vi "Html Title Exchange.vi"(8 "font":T3={"font name"="", "font size"=0.0, "bold"=0, "italic"=0, "underline"=0, "strike through"=0, "font color"=16777216} {"font size" format="%0.2f"; "strike through" items=["Strk Unchanged", "Strk Yes", "Strk No"]; "underline" items=["Und Unchanged", "Und Yes", "Und No"]; "italic" items=["Ital Unchanged", "Ital Yes", "Ital No"]; "bold" items=["Bold Unchanged", "Bold Yes", "Bold No"]}) -> (0 "text color (unchanged)":u32(colorbox)=16777216, 2 "font settings":T2={"Charset (-1)"=-1, "Weight (-1)"=-1, "Name"="", "Size"=" "}, 3 "text options":T1)   [LabVIEW 2014]
uses:
  <vilib>/addons/_office/_wordsub.llb/font.ctl
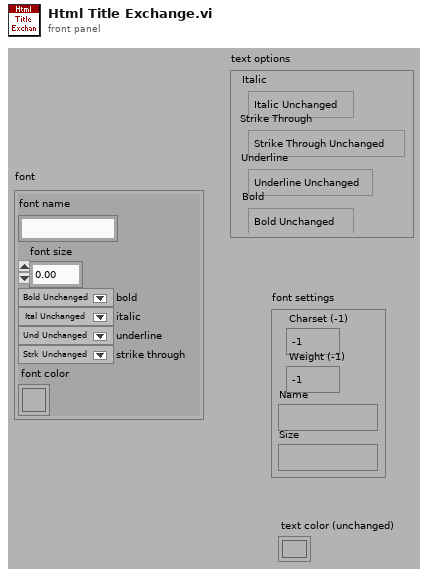
[diagram p1: front panel]
types:
  T1 = cluster{"Italic":enum16{"Italic Unchanged", "Italic On", "Italic Off"}, "Strike Through":enum16{"Strike Through Unchanged", "Strike Through On", "Strike Through Off"}, "Underline":enum16{"Underline Unchanged", "Underline On", "Underline Off"}, "Bold":enum16{"Bold Unchanged", "Bold On", "Bold Off"}}
  T2 = cluster{"Charset (-1)":i16, "Weight (-1)":i16, "Name":string, "Size":string}
  T3 = typedef "font.ctl" = cluster{"font name":string, "font size":dbl, "bold":u16, "italic":u16, "underline":u16, "strike through":u16, "font color":u32}
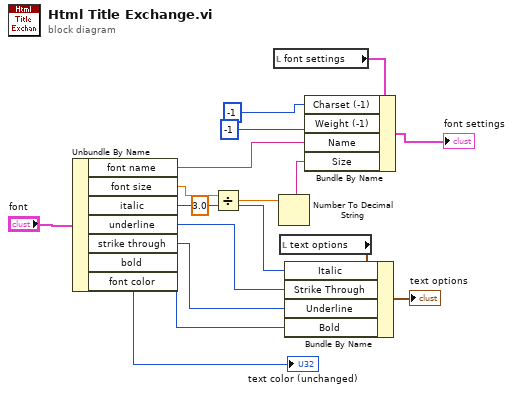
[diagram p0: block diagram]
diagram:
  n1 = Unbundle By Name("font") -> ("font name"=w7:string, "font size"=w3:dbl, "italic"=w15:u16, "underline"=w12:u16, "strike through"=w13:u16, "bold"=w14:u16, "font color"=→"text color (unchanged)":u32)
  n2 = Divide(x=w3, y=3.0) -> (x/y=w1:dbl)
  n3 = local read "font settings"() -> (w9:T2)
  n4 = Number To Decimal String(number=w1) -> (decimal integer string=w6:string)  [unwired: 1 in]
  n5 = local read "text options"() -> (w16:T1)
  n6 = Bundle By Name(cluster=w16, "Italic"=w15, "Strike Through"=w12, "Underline"=w13, "Bold"=w14) -> (→"text options":T1)
  n7 = Bundle By Name(cluster=w9, "Charset (-1)"=i16 -1, "Weight (-1)"=i16 -1, "Name"=w7, "Size"=w6) -> (→"font settings":T2)
